vi "Start Module.vi"(8 "error in (no error)":errorcluster, 11 "TemplateAPI in":refnum<class "ExampleAPI.lvclass">) -> (0 "error out":errorcluster, 1 "Wait for Event Sync?":bool, 2 "Template Broadcast Events":T1, 3 "TemplateAPI out":refnum<class "ExampleAPI.lvclass">, 5 "Module Was Already Running?":bool)   [LabVIEW 2018]
uses:
  4c94efee-2ba9-4b86-bf77-9303cd5a5534.vi
  ExampleAPI.lvclass
  Libraries/Example/Did Init Argument--cluster.ctl
  Libraries/Example/Example.lvlib
  Libraries/Example/Status Updated Argument--cluster.ctl
  Libraries/Example/Error Reported Argument--cluster.ctl
  Libraries/Example/Do Something Argument--cluster.ctl
  Libraries/Example/Stop Argument--cluster.ctl
  Libraries/Example/Get Module Execution Status Argument--cluster.ctl
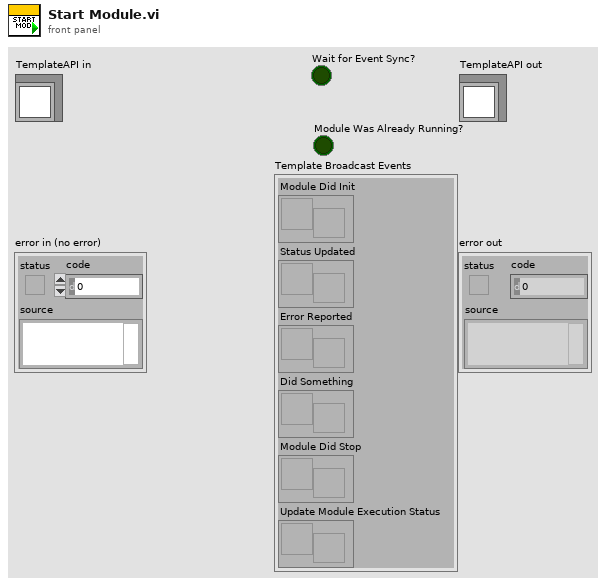
[diagram p1: front panel]
types:
  T1 = cluster{"Module Did Init":refnum<user-event>, "Status Updated":refnum<user-event>, "Error Reported":refnum<user-event>, "Did Something":refnum<user-event>, "Module Did Stop":refnum<user-event>, "Update Module Execution Status":refnum<user-event>}
  T2 = typedef "Template.lvlib/Broadcast Events--cluster.ctl" = cluster{"Module Did Init":refnum<user-event>, "Status Updated":refnum<user-event>, "Error Reported":refnum<user-event>, "Did Something":refnum<user-event>, "Module Did Stop":refnum<user-event>, "Update Module Execution Status":refnum<user-event>}
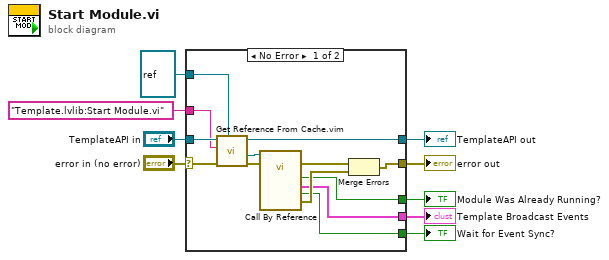
[diagram p0: block diagram]
diagram:
  n1 = case shown="No Error" "error in (no error)" {
    selector: "error in (no error)" -> [w18 w24]
    tunnel: [w16 w24] -> w8
    tunnel: [w21 w23] -> w6
    tunnel: "TemplateAPI in" -> [w22 w23]
    tunnel: "Template.lvlib:Start Module.vi" ("VIQualifiedName") -> [w14 _]
    tunnel: refnum<vi> refnum ("type specifier VI Refnum (for type only)") -> [w13 _]
    tunnel: [w12 _] -> w3
    tunnel: [w11 _] -> w2
    tunnel: [w10 _] -> w1
    frame No Error {
      n2 = call "Get Reference From Cache.vim"("type specifier VI Refnum (for type only)"=w13, "error in (no error)"=w18, "VIQualifiedName"=w14, "App Control API in"=w22) -> ("error out"=w19:errorcluster, "VIRef"=w20:refnum<vi>, "App Control API out"=w21:refnum<class "ExampleAPI.lvclass">)  [unwired: 5 in]
      n3 = call-by-ref "?"(reference=w20, error in=w19) -> (error out=w17:errorcluster, 0:"error out"=w15:errorcluster, "Wait for Event Sync?"=w10:bool, "Template Broadcast Events"=w11:T2, "Module Was Already Running?"=w12:bool)  [unwired: 8 in, 1 out]
      n4 = Merge Errors(w17, w15) -> (w16:errorcluster)
    }
    frame Error {
    }
  }
  "error out" <- w8
  "TemplateAPI out" <- w6
  "Module Was Already Running?" <- w3
  "Template Broadcast Events" <- w2
  "Wait for Event Sync?" <- w1
